vi "Destroy.vi"(8 "error in (no error)":errorcluster, 11 "reference in":refnum<class "PerformanceTest.lvclass">) -> (0 "error out":errorcluster, 3 "reference out":refnum<class "PerformanceTest.lvclass">)   [LabVIEW 2018, in "PerformanceTest.lvclass"]
uses:
  PerformanceTest.lvclass
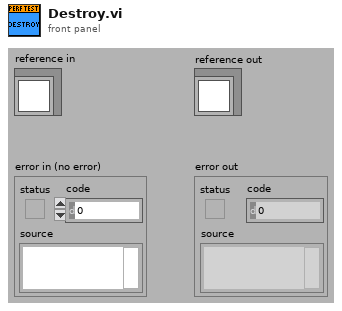
[diagram p1: front panel]
types:
  T1 = typedef "PerformanceTest.lvclass/ObjectAttributes.ctl" = cluster{"Value":dbl}
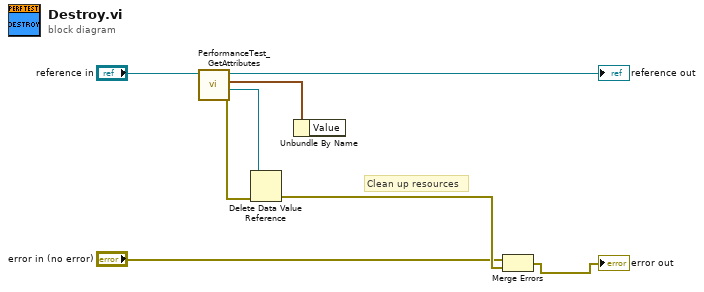
[diagram p0: block diagram]
diagram:
  # "Clean up resources"
  n1 = call "PerformanceTest_GetAttributes.vi"("reference in"="reference in") -> ("error out"=w7:errorcluster, "DataRef"=w6:refnum<data-value>, "Data"=w5:T1, "reference out"=→"reference out":refnum<class "PerformanceTest.lvclass">)  [unwired: 7 in]
  n2 = Delete Data Value Reference(data value reference=w6, error in=w7) -> (error out=w4:errorcluster)  [unwired: 1 out]
  n3 = Unbundle By Name(w5) -> ()  [unwired: 1 out]
  n4 = Merge Errors("error in (no error)", w4) -> (→"error out":errorcluster)
